vi "Image Array to TIFF.vi"(8 "error in":errorcluster, 9 "Data Array":string[](array[string]), 10 "Image Array":T1[](array[plugin-control]), 11 "Destination Image File":path) -> (0 "error out":errorcluster)   [LabVIEW 2012]
uses:
  C:/Users/Andrew/Documents/Apatite to Zircon/AVI Conversion/BitmapsToTIFF.dll
  BitmapsToTIFF.dll
  <vilib>/Utility/file.llb/Write To Spreadsheet File (string).vi
panel:
  out "Base File":string
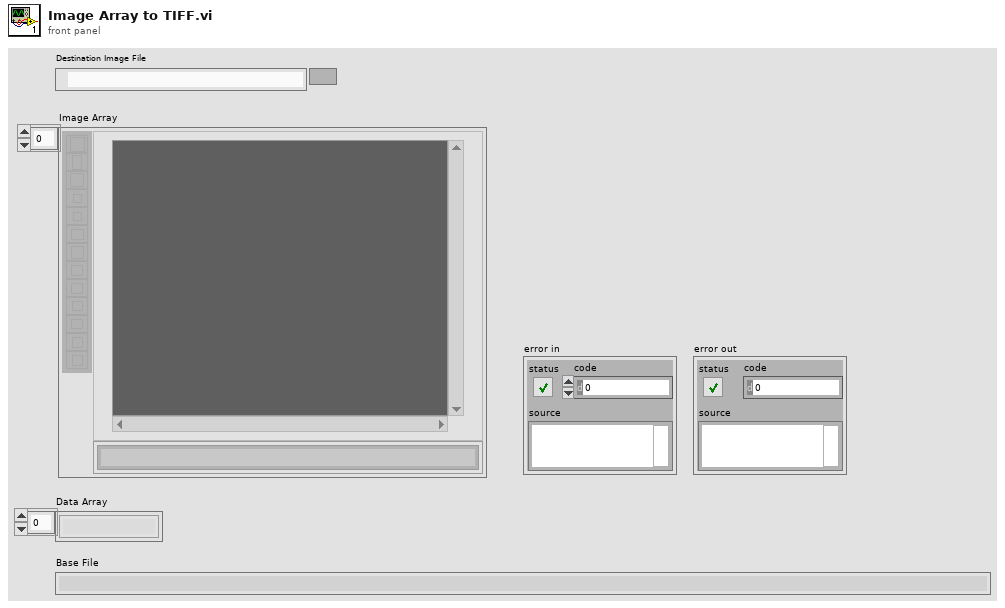
[diagram p1: front panel]
types:
  T1 = typedef "IMAQ Image.ctl" = refnum<image>
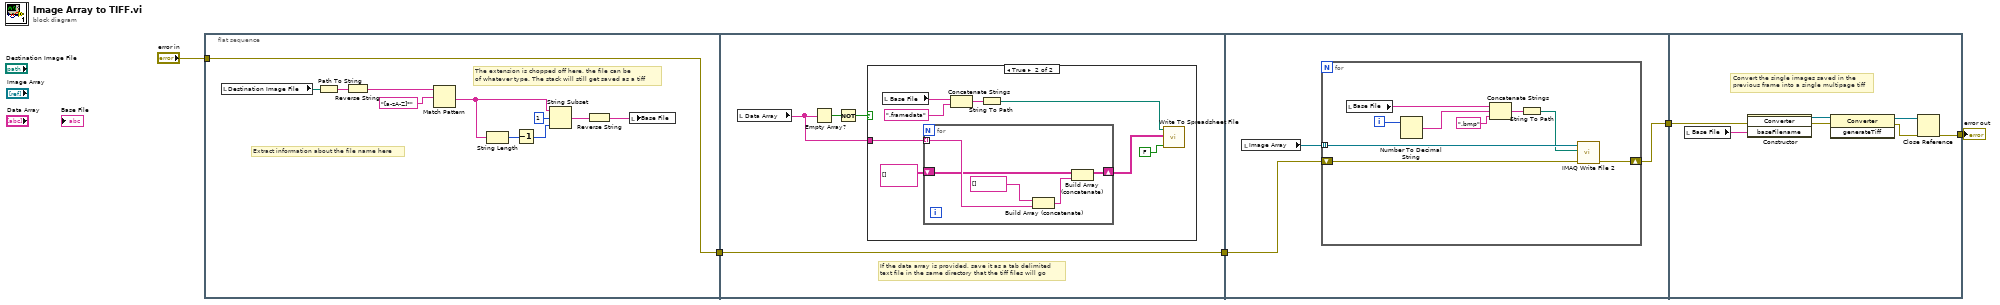
[diagram p0: block diagram]
diagram:
  n1 = flat-sequence {
    tunnel: [w7] -> w4
    tunnel: "error in" -> [w7]
    tunnel: [w17] -> w5
    tunnel: w4 -> [w17]
    tunnel: w5 -> [w35]
    tunnel: [w34] -> w2
    tunnel: w2 -> [w51]
    tunnel: [w46] -> w1
    frame #0 {
      # "The extension is chopped off here, the file can be \nof whatever type. The stack will still get saved as a tiff"
      # "Extract information about the file name here"
      n2 = local read "Destination Image File"() -> (w15:path)
      n3 = Path To String(path=w15) -> (string=w16:string)
      n4 = Reverse String(1:w16) -> (0:w6:string)
      n5 = Match Pattern(string=w6, regular expression="[a-zA-Z]*") -> (after substring=w8:string)  [unwired: 1 in, 3 out]
      n6 = String Length(string=w8) -> (length=w11:i32)
      n7 = Decrement(x=w11) -> (x-1=w10:i32)
      n8 = String Subset(string=w8, offset (0)=1, length (rest)=w10) -> (substring=w9:string)
      n9 = Reverse String(1:w9) -> (0:w13:string)
      n10 = local write "Base File"(w13) -> ()
    }
    frame #1 {
      # "If the data array is provided, save it as a tab delimited\ntext file in the same directory that the tiff files will go"
      n11 = local read "Data Array"() -> (w18:string[])
      n12 = Empty Array?(array=w18) -> (empty?=w20:bool)
      n13 = Not(x=w20) -> (.not. x?=w19:bool)
      n14 = case shown="True" w19 {
        tunnel: w18 -> [_ w23]
        frame False {
        }
        frame True {
          n15 = local read "Base File"() -> (w27:string)
          n16 = for {
            tunnel: w23 -> [w32] mode=indexing
            shift-right: [w31] -> w21
            shift-left: string[][] [] -> [w30]
            n17 = Build Array (concatenate)(string[] [] ("appended array"), w32) -> (w33:string[])
            n18 = Build Array (concatenate)(w30, w33) -> (w31:string[][])
          }
          n19 = Concatenate Strings(w27, ".framedata" ("string")) -> (w25:string)
          n20 = String To Path(string=w25) -> (path=w24:path)
          n21 = call-poly <vilib>:"Write To Spreadsheet File.vi"("append to file? (new file:F)"=FALSE, "2D data"=w21, "file path (dialog if empty)"=w24) -> ()  [unwired: 5 in, 1 out]
        }
      }
    }
    frame #2 {
      n22 = local read "Image Array"() -> (w36:T1[])
      n23 = for {
        tunnel: w36 -> [w45] mode=indexing
        shift-right: [w43] -> w34
        shift-left: w35 -> [w44]
        i -> [w42]
        n24 = local read "Base File"() -> (w39:string)
        n25 = Number To Decimal String(number=w42) -> (decimal integer string=w41:string)  [unwired: 1 in]
        n26 = Concatenate Strings(w39, w41, ".bmp" ("string")) -> (w38:string)
        n27 = String To Path(string=w38) -> (path=w37:path)
        n28 = call-poly "IMAQ Write File 2"("error in (no error)"=w44, "File Path"=w37, "Image"=w45) -> ("error out"=w43:errorcluster)  [unwired: 7 in, 1 out]
      }
    }
    frame #3 {
      # "Convert the single images saved in the \nprevious frame into a single multipage tiff"
      n29 = local read "Base File"() -> (w52:string)
      n30 = constructor class="Converter"(error in=w51, "baseFilename"=w52) -> (reference out=w49:refnum<k24>, error out=w50:errorcluster)  [unwired: 2 in, 2 out]
      n31 = invoke class="Converter" method="generateTiff"(reference=w49, error in=w50) -> (reference out=w48:refnum<k24>, error out=w47:errorcluster)  [unwired: 1 in, 1 out]
      n32 = Close Reference(reference=w48, error in (no error)=w47) -> (error out=w46:errorcluster)
    }
  }
  "error out" <- w1
